vi "Initialize from PS.vi"(8 "error in (no error)":errorcluster, 11 "PS Driver in":refnum<class "PS Driver.lvclass">) -> (0 "error out":errorcluster, 2 "PS Values":T1, 3 "PS Driver out":refnum<class "PS Driver.lvclass">)   [LabVIEW 2020, in "PS Driver.lvlib" / "PS Driver.lvclass"]
uses:
  PS Driver.lvclass
  PS Driver.lvclass/PS Driver.ctl
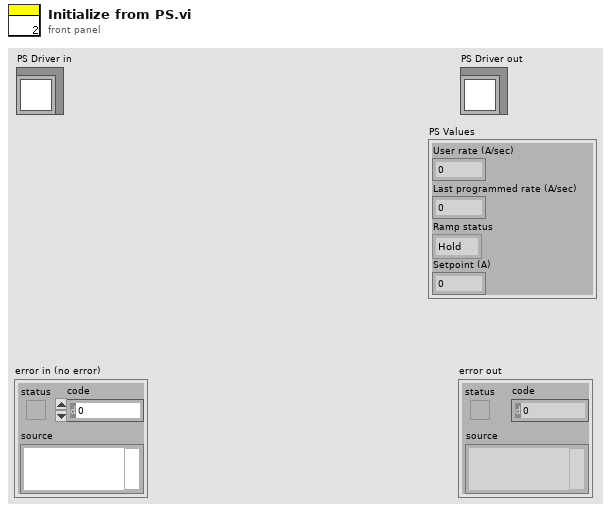
[diagram p1: front panel]
types:
  T1 = cluster{"User rate (A/sec)":dbl, "Last programmed rate (A/sec)":dbl, "Ramp status":enum16{"Hold", "Ramp to zero", "Ramp to setpoint"}, "Setpoint (A)":dbl}
  T2 = cluster{"User rate (T/min)":dbl, "Last programmed rate (T/min)":dbl, "Ramp status":enum16{"Hold", "Ramp to zero", "Ramp to setpoint"}, "Setpoint (T)":dbl}
  T3 = enum16{"Hold", "Ramp to zero", "Ramp to setpoint"}
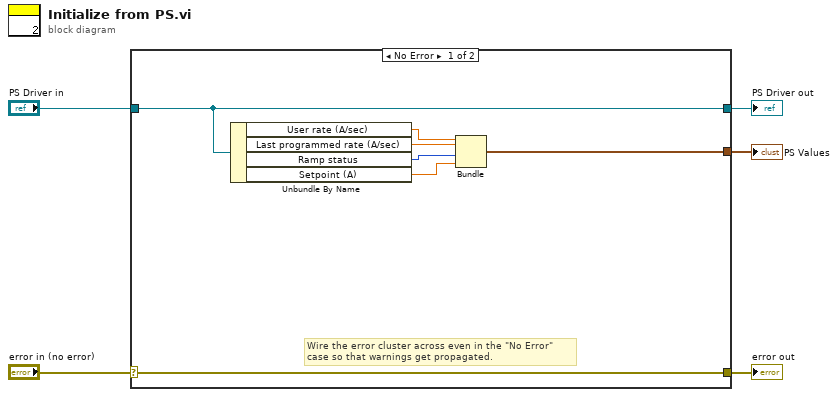
[diagram p0: block diagram]
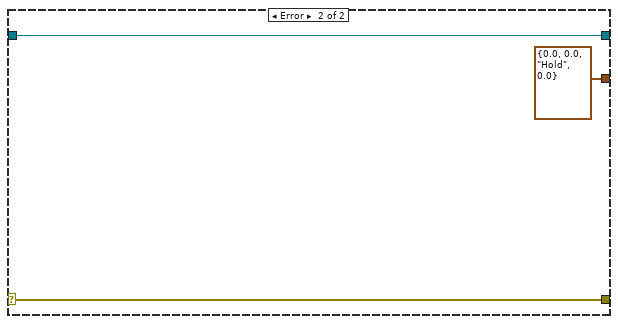
[diagram p2: hidden frame]
diagram:
  n1 = case shown="No Error" "error in (no error)" {
    selector: "error in (no error)" -> [w12 w15]
    tunnel: [w12 w15] -> w4
    tunnel: [w11 w14] -> w2
    tunnel: "PS Driver in" -> [w11 w14]
    tunnel: [w6 T2 {"User rate (T/min)"=0.0, "Last programmed rate (T/min)"=0.0, "Ramp status"=enum."Hold", "Setpoint (T)"=0.0}] -> w1
    frame No Error {
      # "Wire the error cluster across even in the \"No Error\"\ncase so that warnings get propagated."
      n2 = Unbundle By Name(w11) -> ("User rate (A/sec)"=w10:dbl, "Last programmed rate (A/sec)"=w9:dbl, "Ramp status"=w8:T3, "Setpoint (A)"=w7:dbl)
      n3 = Bundle("User rate (A/sec)"=w10, "Last programmed rate (A/sec)"=w9, "Ramp status"=w8, "Setpoint (A)"=w7) -> (w6:T1)  [unwired: 1 in]
    }
    frame Error {
    }
  }
  "error out" <- w4
  "PS Driver out" <- w2
  "PS Values" <- w1
